vi "加标回收调试界面.vi"() -> ()   [LabVIEW 2016, in "质控单元V2.lvlib"]
uses:
  <vilib>/Utility/miscctls.llb/LVPointTypeDef.ctl
  <vilib>/Utility/miscctls.llb/LVPositionTypeDef.ctl
panel:
  in  "关闭":bool
  out "流程 2":T1 {"进样流程"."进样流程-进样"."步骤二："."功能" items=["加标", "进样", "排液", "搅拌", "定量", "延时"]; "进样流程"."进样流程-进样"."步骤一："."功能" items=["加标", "进样", "排液", "搅拌", "定量", "延时"]; "进样流程"."进样流程-进样"."步骤四："."功能" items=["加标", "进样", "排液", "搅拌", "定量", "延时"]; "进样流程"."进样流程-进样"."步骤三："."功能" items=["加标", "进样", "排液", "搅拌", "定量", "延时"]; "进样流程"."进样流程-进样"."步骤六："."功能" items=["加标", "进样", "排液", "搅拌", "定量", "延时"]; "进样流程"."进样流程-进样"."步骤五："."功能" items=["加标", "进样", "排液", "搅拌", "定量", "延时"]; "进样流程"."进样流程-进样"."步骤八："."功能" items=["加标", "进样", "排液", "搅拌", "定量", "延时"]; "进样流程"."进样流程-进样"."步骤七："."功能" items=["加标", "进样", "排液", "搅拌", "定量", "延时"]; "进样流程"."进样流程-进样"."步骤十："."功能" items=["加标", "进样", "排液", "搅拌", "定量", "延时"]; "进样流程"."进样流程-进样"."步骤九："."功能" items=["加标", "进样", "排液", "搅拌", "定量", "延时"]; "进样流程"."进样流程-润洗"."步骤二："."功能" items=["加标", "进样", "排液", "搅拌", "定量", "延时"]; "进样流程"."进样流程-润洗"."步骤一："."功能" items=["加标", "进样", "排液", "搅拌", "定量", "延时"]; "进样流程"."进样流程-润洗"."步骤四："."功能" items=["加标", "进样", "排液", "搅拌", "定量", "延时"]; "进样流程"."进样流程-润洗"."步骤三："."功能" items=["加标", "进样", "排液", "搅拌", "定量", "延时"]; "进样流程"."进样流程-润洗"."步骤六："."功能" items=["加标", "进样", "排液", "搅拌", "定量", "延时"]; "进样流程"."进样流程-润洗"."步骤五："."功能" items=["加标", "进样", "排液", "搅拌", "定量", "延时"]; "进样流程"."进样流程-润洗"."步骤八："."功能" items=["加标", "进样", "排液", "搅拌", "定量", "延时"]; "进样流程"."进样流程-润洗"."步骤七："."功能" items=["加标", "进样", "排液", "搅拌", "定量", "延时"]; "进样流程"."进样流程-润洗"."步骤十："."功能" items=["加标", "进样", "排液", "搅拌", "定量", "延时"]; "进样流程"."进样流程-润洗"."步骤九："."功能" items=["加标", "进样", "排液", "搅拌", "定量", "延时"]; "排液流程"."步骤二："."功能" items=["加标", "进样", "排液", "搅拌", "定量", "延时"]; "排液流程"."步骤一："."功能" items=["加标", "进样", "排液", "搅拌", "定量", "延时"]; "排液流程"."步骤四："."功能" items=["加标", "进样", "排液", "搅拌", "定量", "延时"]; "排液流程"."步骤三："."功能" items=["加标", "进样", "排液", "搅拌", "定量", "延时"]; "排液流程"."步骤六："."功能" items=["加标", "进样", "排液", "搅拌", "定量", "延时"]; "排液流程"."步骤五："."功能" items=["加标", "进样", "排液", "搅拌", "定量", "延时"]; "排液流程"."步骤八："."功能" items=["加标", "进样", "排液", "搅拌", "定量", "延时"]; "排液流程"."步骤七："."功能" items=["加标", "进样", "排液", "搅拌", "定量", "延时"]; "排液流程"."步骤十："."功能" items=["加标", "进样", "排液", "搅拌", "定量", "延时"]; "排液流程"."步骤九："."功能" items=["加标", "进样", "排液", "搅拌", "定量", "延时"]; "加标流程"."加标流程-加标"."步骤二："."功能" items=["加标", "进样", "排液", "搅拌", "定量", "延时"]; "加标流程"."加标流程-加标"."步骤一："."功能" items=["加标", "进样", "排液", "搅拌", "定量", "延时"]; "加标流程"."加标流程-加标"."步骤四："."功能" items=["加标", "进样", "排液", "搅拌", "定量", "延时"]; "加标流程"."加标流程-加标"."步骤三："."功能" items=["加标", "进样", "排液", "搅拌", "定量", "延时"]; "加标流程"."加标流程-加标"."步骤六："."功能" items=["加标", "进样", "排液", "搅拌", "定量", "延时"]; "加标流程"."加标流程-加标"."步骤五："."功能" items=["加标", "进样", "排液", "搅拌", "定量", "延时"]; "加标流程"."加标流程-加标"."步骤八："."功能" items=["加标", "进样", "排液", "搅拌", "定量", "延时"]; "加标流程"."加标流程-加标"."步骤七："."功能" items=["加标", "进样", "排液", "搅拌", "定量", "延时"]; "加标流程"."加标流程-加标"."步骤十："."功能" items=["加标", "进样", "排液", "搅拌", "定量", "延时"]; "加标流程"."加标流程-加标"."步骤九："."功能" items=["加标", "进样", "排液", "搅拌", "定量", "延时"]; "加标流程"."加标流程-定量"."步骤二："."功能" items=["加标", "进样", "排液", "搅拌", "定量", "延时"]; "加标流程"."加标流程-定量"."步骤一："."功能" items=["加标", "进样", "排液", "搅拌", "定量", "延时"]; "加标流程"."加标流程-定量"."步骤四："."功能" items=["加标", "进样", "排液", "搅拌", "定量", "延时"]; "加标流程"."加标流程-定量"."步骤三："."功能" items=["加标", "进样", "排液", "搅拌", "定量", "延时"]; "加标流程"."加标流程-定量"."步骤六："."功能" items=["加标", "进样", "排液", "搅拌", "定量", "延时"]; "加标流程"."加标流程-定量"."步骤五："."功能" items=["加标", "进样", "排液", "搅拌", "定量", "延时"]; "加标流程"."加标流程-定量"."步骤八："."功能" items=["加标", "进样", "排液", "搅拌", "定量", "延时"]; "加标流程"."加标流程-定量"."步骤七："."功能" items=["加标", "进样", "排液", "搅拌", "定量", "延时"]; "加标流程"."加标流程-定量"."步骤十："."功能" items=["加标", "进样", "排液", "搅拌", "定量", "延时"]; "加标流程"."加标流程-定量"."步骤九："."功能" items=["加标", "进样", "排液", "搅拌", "定量", "延时"]; "加标流程"."加标流程-进样"."步骤二："."功能" items=["加标", "进样", "排液", "搅拌", "定量", "延时"]; "加标流程"."加标流程-进样"."步骤一："."功能" items=["加标", "进样", "排液", "搅拌", "定量", "延时"]; "加标流程"."加标流程-进样"."步骤四："."功能" items=["加标", "进样", "排液", "搅拌", "定量", "延时"]; "加标流程"."加标流程-进样"."步骤三："."功能" items=["加标", "进样", "排液", "搅拌", "定量", "延时"]; "加标流程"."加标流程-进样"."步骤六："."功能" items=["加标", "进样", "排液", "搅拌", "定量", "延时"]; "加标流程"."加标流程-进样"."步骤五："."功能" items=["加标", "进样", "排液", "搅拌", "定量", "延时"]; "加标流程"."加标流程-进样"."步骤八："."功能" items=["加标", "进样", "排液", "搅拌", "定量", "延时"]; "加标流程"."加标流程-进样"."步骤七："."功能" items=["加标", "进样", "排液", "搅拌", "定量", "延时"]; "加标流程"."加标流程-进样"."步骤十："."功能" items=["加标", "进样", "排液", "搅拌", "定量", "延时"]; "加标流程"."加标流程-进样"."步骤九："."功能" items=["加标", "进样", "排液", "搅拌", "定量", "延时"]; "加标流程"."加标流程-润洗"."步骤二："."功能" items=["加标", "进样", "排液", "搅拌", "定量", "延时"]; "加标流程"."加标流程-润洗"."步骤一："."功能" items=["加标", "进样", "排液", "搅拌", "定量", "延时"]; "加标流程"."加标流程-润洗"."步骤四："."功能" items=["加标", "进样", "排液", "搅拌", "定量", "延时"]; "加标流程"."加标流程-润洗"."步骤三："."功能" items=["加标", "进样", "排液", "搅拌", "定量", "延时"]; "加标流程"."加标流程-润洗"."步骤六："."功能" items=["加标", "进样", "排液", "搅拌", "定量", "延时"]; "加标流程"."加标流程-润洗"."步骤五："."功能" items=["加标", "进样", "排液", "搅拌", "定量", "延时"]; "加标流程"."加标流程-润洗"."步骤八："."功能" items=["加标", "进样", "排液", "搅拌", "定量", "延时"]; "加标流程"."加标流程-润洗"."步骤七："."功能" items=["加标", "进样", "排液", "搅拌", "定量", "延时"]; "加标流程"."加标流程-润洗"."步骤十："."功能" items=["加标", "进样", "排液", "搅拌", "定量", "延时"]; "加标流程"."加标流程-润洗"."步骤九："."功能" items=["加标", "进样", "排液", "搅拌", "定量", "延时"]}
  in  "请选择模块":T2(radio)=enum."氨氮"
  in  "关于":bool
  in  "Tab Control 4":enum32{"参数"}(tab)
  out "剩余时间":string
  out "当前步骤":string
  out "当前流程":string
  out "告警状态":string
  out "液位状态":string
  out "运行状态":string
  out "通讯状态":bool caption="状态"
  in  "Tab Control 3":enum32{"参数设置", "单步调试", "流程写入"}(tab)
  in  "加标体积读取":bool
  in  "加标体积写入":bool
  in  "蠕动泵参数读取":bool
  in  "蠕动泵参数写入":bool
  in  "B":sgl
  in  "K":sgl
  in  "蠕动泵最小频率(Hz)":sgl
  in  "蠕动泵最大频率(Hz)":sgl
  in  "加标体积(mL)":sgl
  in  "注射泵系数读取":bool
  in  "注射泵系数写入":bool
  in  "蠕动泵2停止":bool
  in  "蠕动泵2正转":bool
  in  "蠕动泵2反转":bool
  in  "蠕动泵1停止":bool
  in  "蠕动泵1正转":bool
  in  "蠕动泵1反转":bool
  in  "三通阀2打开":bool
  in  "三通阀2关闭":bool
  in  "三通阀1打开":bool
  in  "三通阀1关闭":bool
  in  "注射泵复位":bool
  in  "注射泵暂停":bool
  in  "注射泵注入量":sgl=1000.0 min=0 max=1000 format="%u μL"
  in  "注射泵注出量":sgl=1000.0 min=0 max=1000 format="%u μL"
  in  "注射泵注出":bool
  in  "注射泵注入":bool
  in  "三通阀打开":bool
  in  "三通阀关闭":bool
  in  "流程保存":bool
  in  "流程加载":bool
  in  "流程写入":bool
  in  "流程读取":bool
  in  "子流程":u16(ring) items=["润洗"]
  in  "主流程":enum16{"进样流程", "加标流程", "排液流程"}(ring)
  in  "流程":T3 {"步骤二："."功能" items=["加标", "进样", "排液", "搅拌", "定量", "延时"]; "步骤四："."功能" items=["加标", "进样", "排液", "搅拌", "定量", "延时"]; "步骤六："."功能" items=["加标", "进样", "排液", "搅拌", "定量", "延时"]; "步骤八："."功能" items=["加标", "进样", "排液", "搅拌", "定量", "延时"]; "步骤十："."功能" items=["加标", "进样", "排液", "搅拌", "定量", "延时"]; "步骤一："."功能" items=["加标", "进样", "排液", "搅拌", "定量", "延时"]; "步骤三："."功能" items=["加标", "进样", "排液", "搅拌", "定量", "延时"]; "步骤五："."功能" items=["加标", "进样", "排液", "搅拌", "定量", "延时"]; "步骤七："."功能" items=["加标", "进样", "排液", "搅拌", "定量", "延时"]; "步骤九："."功能" items=["加标", "进样", "排液", "搅拌", "定量", "延时"]}
  in  "Tab Control 2":enum32{"参数"}(tab)
  in  "组合操作加标":bool
  in  "启动进样流程":bool
  in  "启动加标流程":bool
  in  "启动排液流程":bool
  in  "停止所有流程":bool
  in  "组合操作停止":bool
  in  "组合操作定量":bool
  in  "组合操作进空气":bool
  in  "组合操作排废液":bool
  in  "组合操作进水样":bool
  in  "清除告警":bool
  in  "加标体积输入":sgl=0.1 min=0 max=1000 format="%#.4f mL"
  # "仪器状态"
  # "柱塞泵泵系数"
  # "柱塞泵"
  # "三通阀"
  # "泵阀"
  # "三通阀1"
  # "三通阀2"
  # "蠕动泵1"
  # "蠕动泵2"
  # "仪器端："
  # "PC端："
  # "组合步骤"
  # "测试流程"
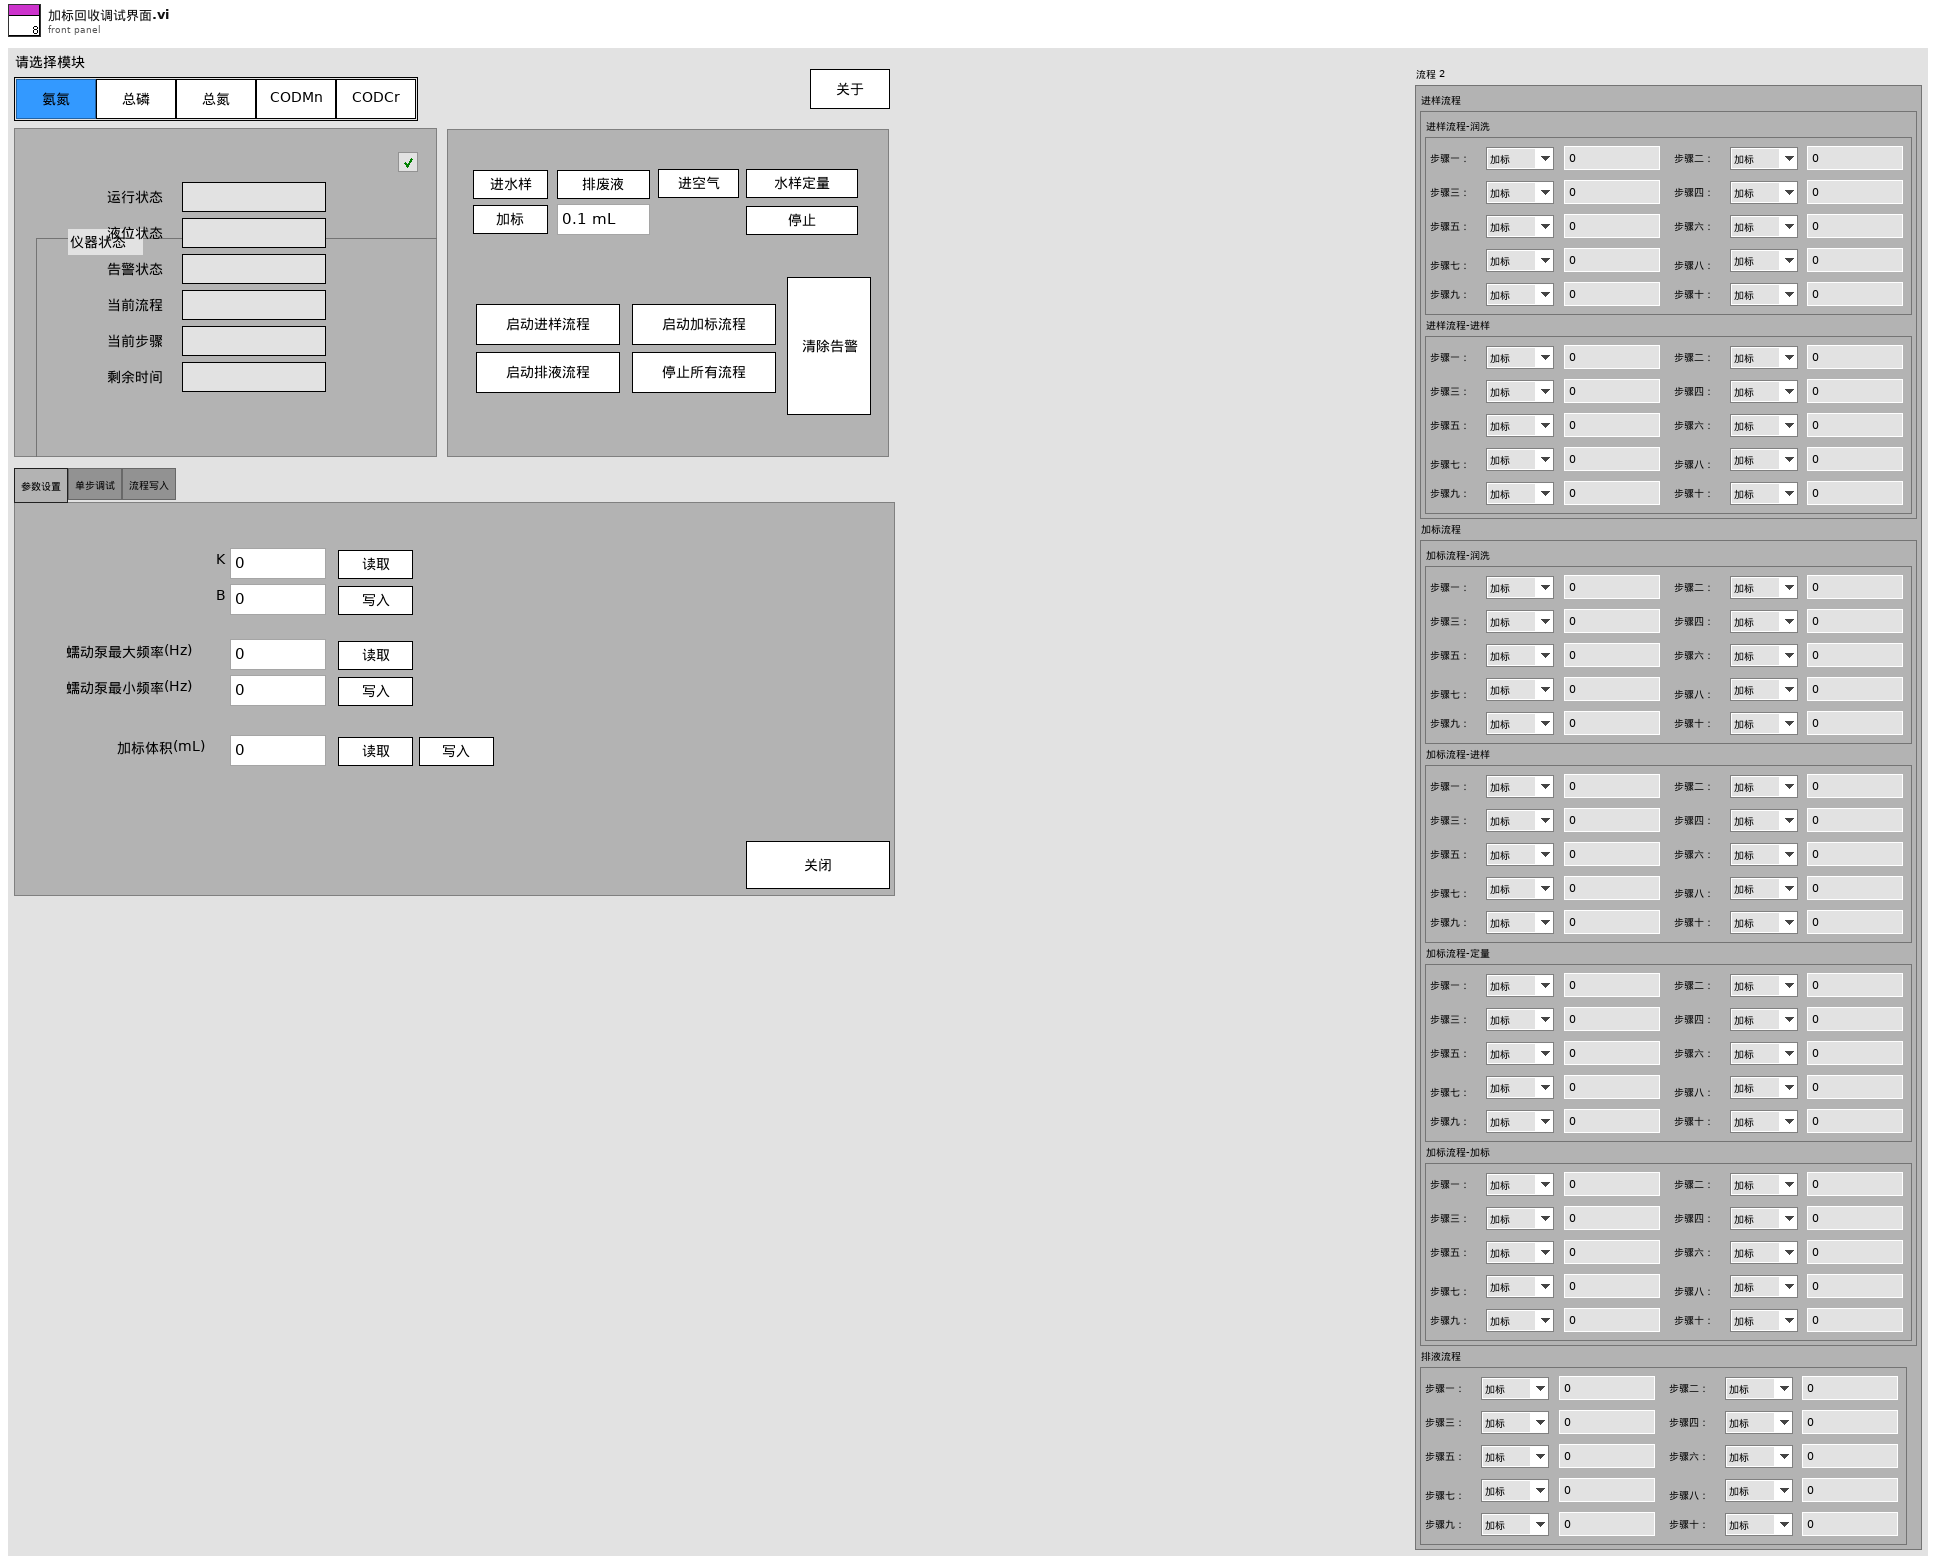
[diagram p1: front panel]
types:
  T1 = cluster{"进样流程":cluster{"进样流程-润洗":cluster{"步骤一：":cluster{"功能":u16, "值":sgl}, "步骤二：":cluster{"功能":u16, "值":sgl}, "步骤三：":cluster{"功能":u16, "值":sgl}, "步骤四：":cluster{"功能":u16, "值":sgl}, "步骤五：":cluster{"功能":u16, "值":sgl}, "步骤六：":cluster{"功能":u16, "值":sgl}, "步骤七：":cluster{"功能":u16, "值":sgl}, "步骤八：":cluster{"功能":u16, "值":sgl}, "步骤九：":cluster{"功能":u16, "值":sgl}, "步骤十：":cluster{"功能":u16, "值":sgl}}, "进样流程-进样":cluster{"步骤一：":cluster{"功能":u16, "值":sgl}, "步骤二：":cluster{"功能":u16, "值":sgl}, "步骤三：":cluster{"功能":u16, "值":sgl}, "步骤四：":cluster{"功能":u16, "值":sgl}, "步骤五：":cluster{"功能":u16, "值":sgl}, "步骤六：":cluster{"功能":u16, "值":sgl}, "步骤七：":cluster{"功能":u16, "值":sgl}, "步骤八：":cluster{"功能":u16, "值":sgl}, "步骤九：":cluster{"功能":u16, "值":sgl}, "步骤十：":cluster{"功能":u16, "值":sgl}}}, "加标流程":cluster{"加标流程-润洗":cluster{"步骤一：":cluster{"功能":u16, "值":sgl}, "步骤二：":cluster{"功能":u16, "值":sgl}, "步骤三：":cluster{"功能":u16, "值":sgl}, "步骤四：":cluster{"功能":u16, "值":sgl}, "步骤五：":cluster{"功能":u16, "值":sgl}, "步骤六：":cluster{"功能":u16, "值":sgl}, "步骤七：":cluster{"功能":u16, "值":sgl}, "步骤八：":cluster{"功能":u16, "值":sgl}, "步骤九：":cluster{"功能":u16, "值":sgl}, "步骤十：":cluster{"功能":u16, "值":sgl}}, "加标流程-进样":cluster{"步骤一：":cluster{"功能":u16, "值":sgl}, "步骤二：":cluster{"功能":u16, "值":sgl}, "步骤三：":cluster{"功能":u16, "值":sgl}, "步骤四：":cluster{"功能":u16, "值":sgl}, "步骤五：":cluster{"功能":u16, "值":sgl}, "步骤六：":cluster{"功能":u16, "值":sgl}, "步骤七：":cluster{"功能":u16, "值":sgl}, "步骤八：":cluster{"功能":u16, "值":sgl}, "步骤九：":cluster{"功能":u16, "值":sgl}, "步骤十：":cluster{"功能":u16, "值":sgl}}, "加标流程-定量":cluster{"步骤一：":cluster{"功能":u16, "值":sgl}, "步骤二：":cluster{"功能":u16, "值":sgl}, "步骤三：":cluster{"功能":u16, "值":sgl}, "步骤四：":cluster{"功能":u16, "值":sgl}, "步骤五：":cluster{"功能":u16, "值":sgl}, "步骤六：":cluster{"功能":u16, "值":sgl}, "步骤七：":cluster{"功能":u16, "值":sgl}, "步骤八：":cluster{"功能":u16, "值":sgl}, "步骤九：":cluster{"功能":u16, "值":sgl}, "步骤十：":cluster{"功能":u16, "值":sgl}}, "加标流程-加标":cluster{"步骤一：":cluster{"功能":u16, "值":sgl}, "步骤二：":cluster{"功能":u16, "值":sgl}, "步骤三：":cluster{"功能":u16, "值":sgl}, "步骤四：":cluster{"功能":u16, "值":sgl}, "步骤五：":cluster{"功能":u16, "值":sgl}, "步骤六：":cluster{"功能":u16, "值":sgl}, "步骤七：":cluster{"功能":u16, "值":sgl}, "步骤八：":cluster{"功能":u16, "值":sgl}, "步骤九：":cluster{"功能":u16, "值":sgl}, "步骤十：":cluster{"功能":u16, "值":sgl}}}, "排液流程":cluster{"步骤一：":cluster{"功能":u16, "值":sgl}, "步骤二：":cluster{"功能":u16, "值":sgl}, "步骤三：":cluster{"功能":u16, "值":sgl}, "步骤四：":cluster{"功能":u16, "值":sgl}, "步骤五：":cluster{"功能":u16, "值":sgl}, "步骤六：":cluster{"功能":u16, "值":sgl}, "步骤七：":cluster{"功能":u16, "值":sgl}, "步骤八：":cluster{"功能":u16, "值":sgl}, "步骤九：":cluster{"功能":u16, "值":sgl}, "步骤十：":cluster{"功能":u16, "值":sgl}}}
  T2 = enum32{"未选择", "氨氮", "总磷", "总氮", "CODMn", "CODCr", "氨氮总磷", "总磷总氮"}
  T3 = cluster{"步骤一：":cluster{"功能":u16, "值":sgl}, "步骤二：":cluster{"功能":u16, "值":sgl}, "步骤三：":cluster{"功能":u16, "值":sgl}, "步骤四：":cluster{"功能":u16, "值":sgl}, "步骤五：":cluster{"功能":u16, "值":sgl}, "步骤六：":cluster{"功能":u16, "值":sgl}, "步骤七：":cluster{"功能":u16, "值":sgl}, "步骤八：":cluster{"功能":u16, "值":sgl}, "步骤九：":cluster{"功能":u16, "值":sgl}, "步骤十：":cluster{"功能":u16, "值":sgl}}
  T4 = typedef "LVPositionTypeDef.ctl" = cluster{"Left":i32, "Top":i32}
  T5 = typedef "LVPointTypeDef.ctl" = cluster{"Horizontal":i16, "Vertical":i16}
  T6 = typedef "质控单元V2.lvlib/质控slave id.ctl" = enum16{"null", "氨氮", "总磷", "总氮", "CODMn", "CODCr"}
  T7 = typedef "质控单元V2.lvlib/质控注射泵操作.ctl" = enum16{"打开三通阀", "关闭三通阀", "注射泵吸入", "注射泵排出", "注射泵暂停", "注射泵复位"}
  T8 = typedef "质控单元V2.lvlib/质控组合命令区.ctl" = enum16{"停止", "进水样", "排废液", "进空气（搅拌）", "定量（反转定量）", "加标"}
  T9 = typedef "质控单元V2.lvlib/质控流程控制.ctl" = enum16{"待机", "启动进样流程", "启动加标流程", "启动排液流程", "停止流程", "加标（单独一步骤）"}
  T10 = typedef "质控单元V2.lvlib/质控仪器状态显示.ctl" = cluster{"运行模式":string, "运行状态":string, "液位状态":string, "告警状态":string, "当前流程":string, "当前步骤":string, "剩余时间":string}
  T11 = typedef "质控单元V2.lvlib/质控蠕动泵操作.ctl" = u16
  T12 = typedef "LVRectTypeDef.ctl" = cluster{"Left":i16, "Top":i16, "Right":i16, "Bottom":i16}
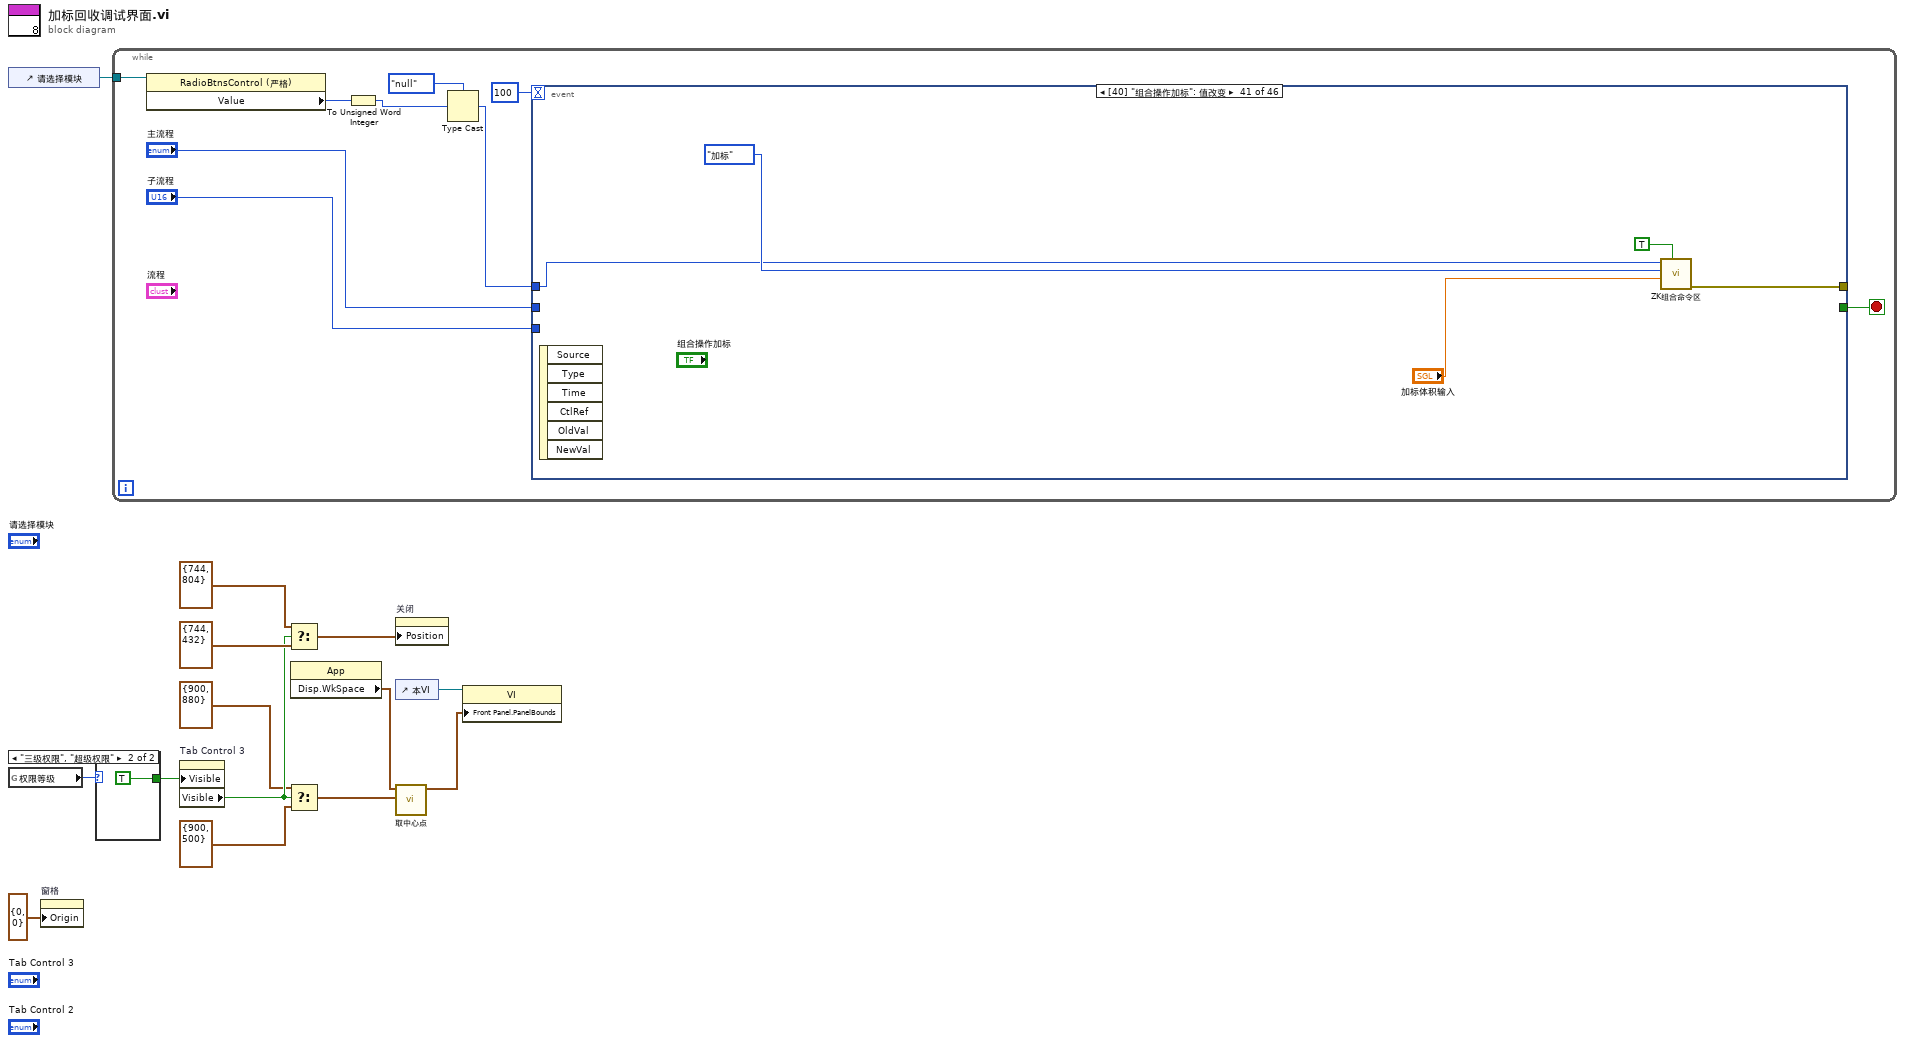
[diagram p0: block diagram]
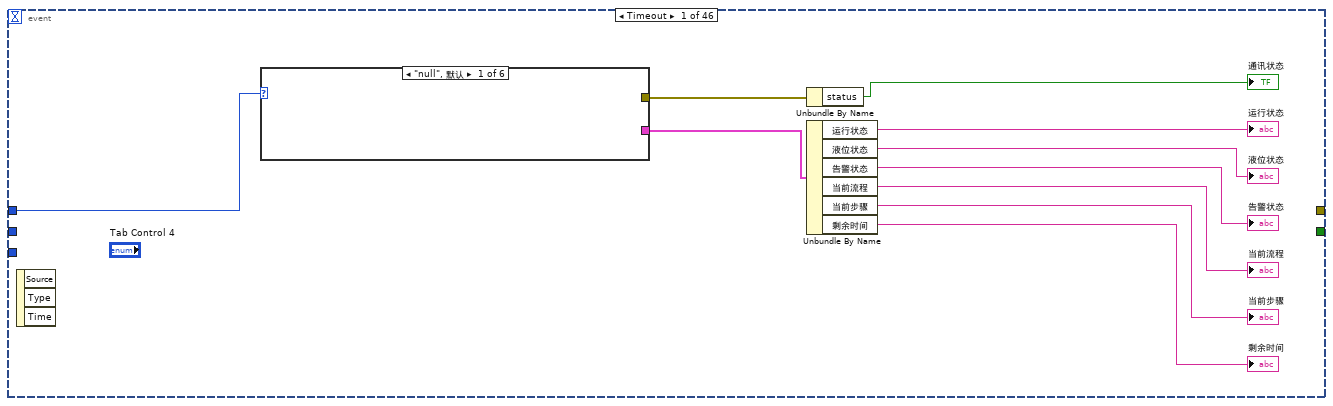
[diagram p3: hidden frame]
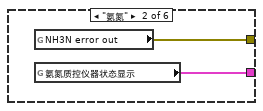
[diagram p4: hidden frame]
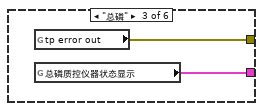
[diagram p5: hidden frame]
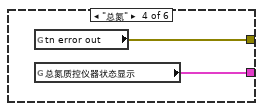
[diagram p6: hidden frame]
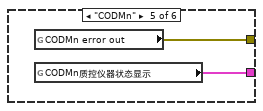
[diagram p7: hidden frame]
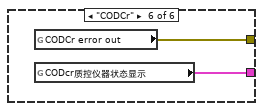
[diagram p8: hidden frame]
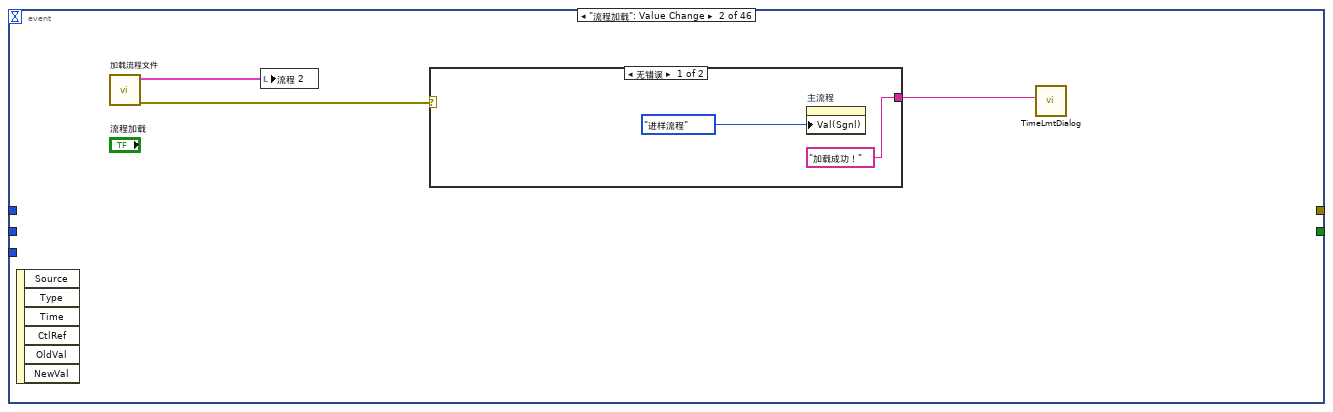
[diagram p9: hidden frame]
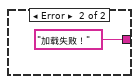
[diagram p10: hidden frame]
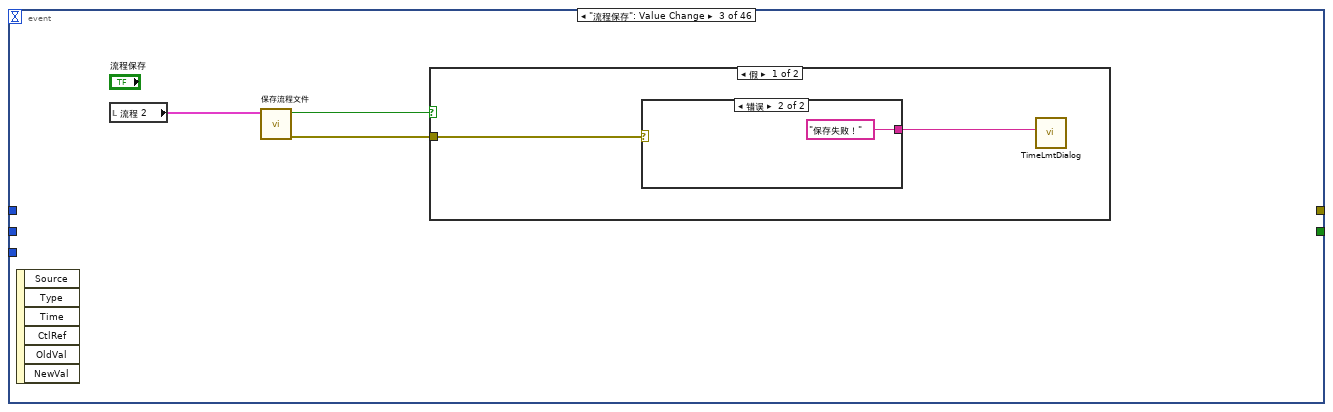
[diagram p11: hidden frame]
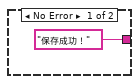
[diagram p12: hidden frame]
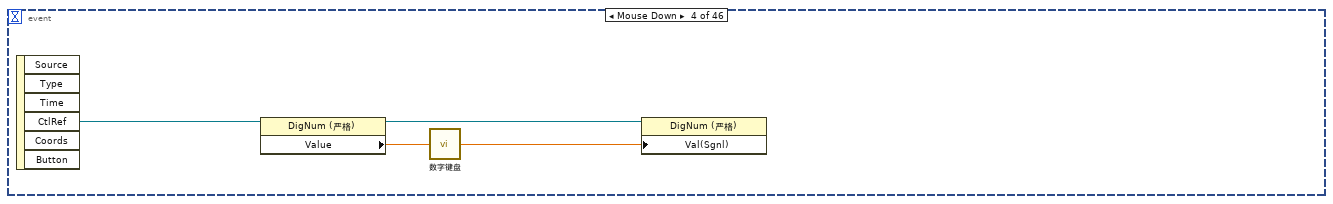
[diagram p14: hidden frame]
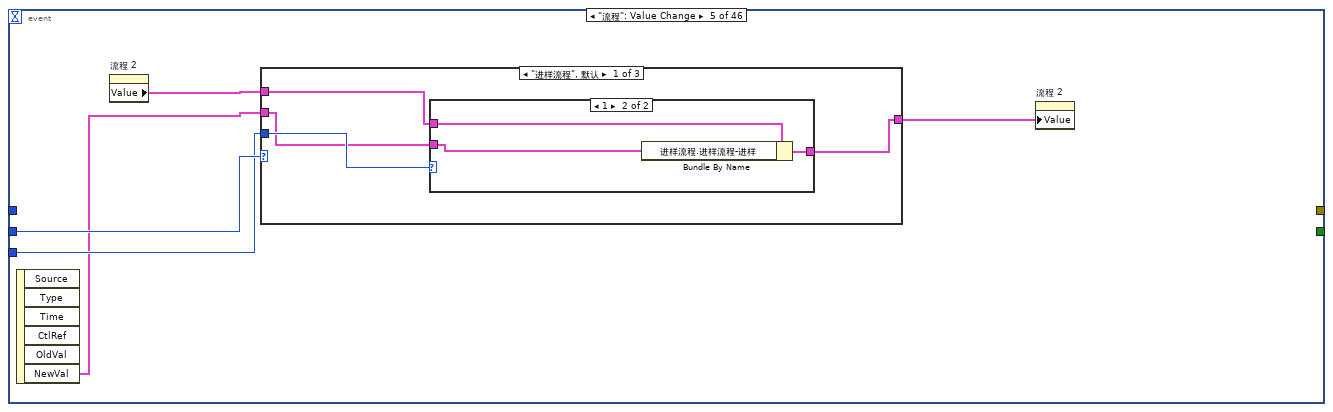
[diagram p15: hidden frame]
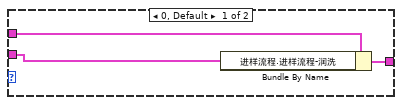
[diagram p16: hidden frame]
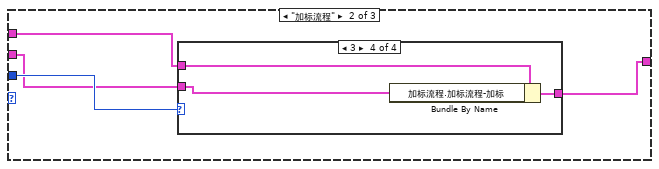
[diagram p17: hidden frame]
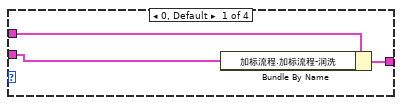
[diagram p18: hidden frame]
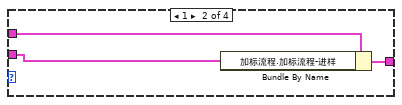
[diagram p19: hidden frame]
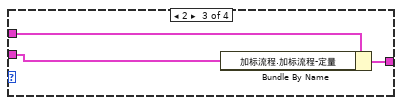
[diagram p20: hidden frame]
diagram:
  n1 = control-ref of="请选择模块"() -> (w13:refnum<vi>)
  n2 = global read "ZK非断电保存全局变量.vi" "权限等级"() -> (w2:enum16{"一级权限", "二级权限", "三级权限", "超级权限"})
  n3 = property on="窗格" class="Pane"("Origin"=T5 {"Horizontal"=0, "Vertical"=0} ("原点")) -> ()  [unwired: 2 in, 2 out]
  n4 = case shown="\"三级权限\", \"超级权限\"" w2 {
    tunnel: [_ TRUE] -> w1
    frame "一级权限", Default {
    }
    frame "三级权限", "超级权限" {
    }
  }
  n5 = while {
    tunnel: w13 -> [w22]
    stop <- w24 stop-if-true
    n6 = property class="RadioBtnsControl (严格)"(reference=w22) -> ("Value"=w19:T2)  [unwired: 1 in, 2 out]
    n7 = To Unsigned Word Integer(number=w19) -> (unsigned 16bit integer=w18:u16)
    n8 = Type Cast(type=质控slave_id."null" ("请选择模块"), x=w18) -> (*(type *) &x=w20:T6)
    n9 = event shown="[40] \"组合操作加标\": 值改变" {
      selector: _ -> [_ _ _ _ _ _ _ _ _ _ _ _ _ _ _ _ _ _ _ _ _ _ _ _ _ _ _ _ _ _ _ _ _ _ _ _ _ _ _ _ _ _ _ _ _ _]
      dyn-events: _ -> [_ _ _ _ _ _ _ _ _ _ _ _ _ _ _ _ _ _ _ _ _ _ _ _ _ _ _ _ _ _ _ _ _ _ _ _ _ _ _ _ _ _ _ _ _ _]
      timeout: 100 -> [_ _ _ _ _ _ _ _ _ _ _ _ _ _ _ _ _ _ _ _ _ _ _ _ _ _ _ _ _ _ _ _ _ _ _ _ _ _ _ _ _ _ _ _ _ _]
      tunnel: [_ _ _ _ _ _ _ _ _ _ _ TRUE _ _ _ _ _ _ _ _ _ _ _ _ _ _ _ _ _ _ _ _ _ _ _ _ _ _ _ _ _ _ _ _ _ _] -> w24
      tunnel: [_ _ _ _ _ _ _ _ _ _ w160 _ _ _ w174 w179 w186 w189 w195 w199 w202 w207 w217 w227 w231 w235 w238 w242 w246 w250 w255 w259 w263 w267 w271 w275 w279 w283 w287 w291 w296 w300 w304 w308 w312 w316] -> _
      tunnel: w20 -> [w27 _ _ _ _ w99 w102 _ _ w157 w158 _ _ _ w172 w177 w182 w187 w192 w196 w200 w204 w210 w221 w228 w232 w236 w240 w244 w248 w252 w256 w260 w264 w268 w272 w276 w280 w284 w288 w293 w297 w301 w305 w309 w313]
      tunnel: "子流程" -> [_ _ _ _ w64 _ _ w108 _ _ _ _ _ _ _ _ _ _ _ _ _ _ _ _ _ _ _ _ _ _ _ _ _ _ _ _ _ _ _ _ _ _ _ _ _ _]
      tunnel: "主流程" -> [_ _ _ _ w65 _ _ _ w134 _ _ _ _ _ _ _ _ _ _ _ _ _ _ _ _ _ _ _ _ _ _ _ _ _ _ _ _ _ _ _ _ _ _ _ _ _]
      event Timeout {
        n10 = event-data() -> ()  [unwired: 1 in, 3 out]
        n11 = case shown="\"null\", 默认" w27 {
          tunnel: [_ w36 w38 w40 w42 w44] -> w34
          tunnel: [_ w35 w37 w39 w41 w43] -> w26
          frame "null", Default {
          }
          frame "氨氮" {
            n12 = global read "ZK非断电保存全局变量.vi" "NH3N error out"() -> (w35:errorcluster)
            n13 = global read "ZK非断电保存全局变量.vi" "氨氮质控仪器状态显示"() -> (w36:T10)
          }
          frame "总磷" {
            n14 = global read "ZK非断电保存全局变量.vi" "tp error out"() -> (w37:errorcluster)
            n15 = global read "ZK非断电保存全局变量.vi" "总磷质控仪器状态显示"() -> (w38:T10)
          }
          frame "总氮" {
            n16 = global read "ZK非断电保存全局变量.vi" "tn error out"() -> (w39:errorcluster)
            n17 = global read "ZK非断电保存全局变量.vi" "总氮质控仪器状态显示"() -> (w40:T10)
          }
          frame "CODMn" {
            n18 = global read "ZK非断电保存全局变量.vi" "CODMn error out"() -> (w41:errorcluster)
            n19 = global read "ZK非断电保存全局变量.vi" "CODMn质控仪器状态显示"() -> (w42:T10)
          }
          frame "CODCr" {
            n20 = global read "ZK非断电保存全局变量.vi" "CODCr error out"() -> (w43:errorcluster)
            n21 = global read "ZK非断电保存全局变量.vi" "CODcr质控仪器状态显示"() -> (w44:T10)
          }
        }
        n22 = Unbundle By Name(w26) -> ("status"=→"通讯状态":bool)
        n23 = Unbundle By Name(w34) -> ("运行状态"=→"运行状态":string, "液位状态"=→"液位状态":string, "告警状态"=→"告警状态":string, "当前流程"=→"当前流程":string, "当前步骤"=→"当前步骤":string, "剩余时间"=→"剩余时间":string)
      }
      event "流程加载": Value Change {
        n24 = event-data() -> ()  [unwired: 1 in, 6 out]
        n25 = call "加载流程文件.vi"() -> ("错误输出"=w46:errorcluster, "流程"=w47:T1)  [unwired: 10 in]
        n26 = local write "流程 2"(w47) -> ()
        n27 = case shown="无错误" w46 {
          tunnel: ["加载成功！" "加载失败！"] -> w45
          frame No Error {
            n28 = property on="主流程" class="Enum (严格)"("Val(Sgnl)"=enum16{"进样流程", "加标流程", "排液流程"}."进样流程" ("值(信号)")) -> ()  [unwired: 2 in, 2 out]
          }
          frame Error {
          }
        }
        n29 = call "TimeLmtDialog.vi"("Infoin"=w45) -> ()  [unwired: 11 in]
      }
      event "流程保存": Value Change {
        n30 = event-data() -> ()  [unwired: 1 in, 6 out]
        n31 = local read "流程 2"() -> (w53:T1)
        n32 = call "保存流程文件.vi"("流程"=w53) -> ("错误输出"=w52:errorcluster, "cancelled"=w51:bool)  [unwired: 9 in]
        n33 = case shown="假" w51 {
          tunnel: w52 -> [w54 _]
          frame False {
            n34 = case shown="错误" w54 {
              tunnel: ["保存成功！" "保存失败！"] -> w55
              frame No Error {
              }
              frame Error {
              }
            }
            n35 = call "TimeLmtDialog.vi"("Infoin"=w55) -> ()  [unwired: 11 in]
          }
          frame True {
          }
        }
      }
      event "流程.步骤一：.值", "流程.步骤二：.值", "流程.步骤三：.值", "流程.步骤四：.值", "流程.步骤五：.值", "流程.步骤六：.值", "流程.步骤七：.值", "流程.步骤八：.值", "流程.步骤九：.值", "流程.步骤十：.值": Mouse Down {
        n36 = event-data() -> ("CtlRef"=w58:refnum<vi>)  [unwired: 1 in, 5 out]
        n37 = property class="DigNum (严格)"(reference=w58) -> (reference out=w61:refnum<vi>, "Value"=w59:sgl)  [unwired: 1 in, 1 out]
        n38 = call "数字键盘.vi"("OldNumber"=w59) -> ("NewNumber"=w60:sgl)
        n39 = property class="DigNum (严格)"(reference=w61, "Val(Sgnl)"=w60) -> ()  [unwired: 1 in, 2 out]
      }
      event "流程": Value Change {
        n40 = event-data() -> ("NewVal"=w63:T3)  [unwired: 1 in, 5 out]
        n41 = property on="流程 2" class="Clust (严格)"() -> ("Value"=w66:T1)  [unwired: 2 in, 2 out]
        n42 = case shown="\"进样流程\", 默认" w65 {
          tunnel: w66 -> [w69 w79 w95]
          tunnel: w64 -> [w70 w80 _]
          tunnel: w63 -> [w68 w77 w94]
          tunnel: [w67 w78 w93] -> w62
          frame "进样流程", Default {
            n43 = case shown="1" w70 {
              tunnel: w69 -> [w73 w76]
              tunnel: w68 -> [w72 w75]
              tunnel: [w71 w74] -> w67
              frame 0, Default {
                n44 = Bundle By Name(cluster=w73, "进样流程.进样流程-润洗"=w72) -> (w71:T1)
              }
              frame 1 {
                n45 = Bundle By Name(cluster=w76, "进样流程.进样流程-进样"=w75) -> (w74:T1)
              }
            }
          }
          frame "加标流程" {
            n46 = case shown="3" w80 {
              tunnel: w79 -> [w83 w86 w88 w92]
              tunnel: [w82 w84 w87 w90] -> w78
              tunnel: w77 -> [w81 w85 w89 w91]
              frame 0, Default {
                n47 = Bundle By Name(cluster=w83, "加标流程.加标流程-润洗"=w81) -> (w82:T1)
              }
              frame 1 {
                n48 = Bundle By Name(cluster=w86, "加标流程.加标流程-进样"=w85) -> (w84:T1)
              }
              frame 2 {
                n49 = Bundle By Name(cluster=w88, "加标流程.加标流程-定量"=w89) -> (w87:T1)
              }
              frame 3 {
                n50 = Bundle By Name(cluster=w92, "加标流程.加标流程-加标"=w91) -> (w90:T1)
              }
            }
          }
          frame "排液流程" {
            n51 = Bundle By Name(cluster=w95, "排液流程"=w94) -> (w93:T1)
          }
        }
        n52 = property on="流程 2" class="Clust (严格)"("Value"=w62) -> ()  [unwired: 2 in, 2 out]
      }
      event "流程读取": Value Change {
        n53 = event-data() -> ()  [unwired: 1 in, 6 out]
        n54 = call "ZK流程读取.vi"("是否启用通讯通知"=TRUE, "Slave ID"=w99) -> ("error out"=w96:errorcluster, "流程"=→"流程 2":T1)  [unwired: 8 in]
        n55 = case shown="无错误" w96 {
          frame No Error {
            n56 = property on="主流程" class="Enum (严格)"("Val(Sgnl)"=enum16{"进样流程", "加标流程", "排液流程"}."进样流程" ("值(信号)")) -> ()  [unwired: 2 in, 2 out]
          }
          frame Error {
          }
        }
      }
      event "流程写入": Value Change {
        n57 = event-data() -> ()  [unwired: 1 in, 6 out]
        n58 = property on="流程 2" class="Clust (严格)"() -> ("Value"=w103:T1)  [unwired: 2 in, 2 out]
        n59 = call "ZK流程写入.vi"("是否启用通讯通知"=TRUE, "流程"=w103, "Slave ID"=w102) -> ()  [unwired: 8 in, 1 out]
      }
      event "主流程": Value Change {
        n60 = event-data() -> ("NewVal"=w104:enum16{"进样流程", "加标流程", "排液流程"})  [unwired: 1 in, 5 out]
        n61 = local read "流程 2"() -> (w109:T1)
        n62 = case shown="\"进样流程\", 默认" w104 {
          tunnel: w109 -> [w112 w120 w132]
          tunnel: w108 -> [w113 w121 _]
          tunnel: [w111 w119 w131] -> w107
          tunnel: [string[] ["润洗", "进样"] ("字符串[]") string[] ["润洗", "进样", "定量", "加标"] ("字符串[]") string[] ["排液"] ("字符串[]")] -> w106
          frame "进样流程", Default {
            n63 = case shown="0, 默认" w113 {
              tunnel: w112 -> [w115 w117]
              tunnel: [w114 w116] -> w111
              frame 0, Default {
                n64 = Unbundle By Name(w115) -> ("进样流程.进样流程-润洗"=w114:T3)
              }
              frame 1 {
                n65 = Unbundle By Name(w117) -> ("进样流程.进样流程-进样"=w116:T3)
              }
            }
          }
          frame "加标流程" {
            n66 = case shown="3" w121 {
              tunnel: w120 -> [w123 w125 w127 w129]
              tunnel: [w122 w124 w126 w128] -> w119
              frame 0, Default {
                n67 = Unbundle By Name(w123) -> ("加标流程.加标流程-润洗"=w122:T3)
              }
              frame 1 {
                n68 = Unbundle By Name(w125) -> ("加标流程.加标流程-进样"=w124:T3)
              }
              frame 2 {
                n69 = Unbundle By Name(w127) -> ("加标流程.加标流程-定量"=w126:T3)
              }
              frame 3 {
                n70 = Unbundle By Name(w129) -> ("加标流程.加标流程-加标"=w128:T3)
              }
            }
          }
          frame "排液流程" {
            n71 = Unbundle By Name(w132) -> ("排液流程"=w131:T3)
          }
        }
        n72 = local write "流程"(w107) -> ()
        n73 = property on="子流程" class="Ring (严格)"("Strings []"=w106, "Value"=0) -> ()  [unwired: 2 in, 2 out]
      }
      event "子流程": Value Change {
        n74 = event-data() -> ("NewVal"=w133:u16)  [unwired: 1 in, 5 out]
        n75 = local read "流程 2"() -> (w136:T1)
        n76 = case shown="\"进样流程\", 默认" w134 {
          tunnel: w136 -> [w138 w145 w156]
          tunnel: w133 -> [w139 w146 _]
          tunnel: [w137 w144 w155] -> w135
          frame "进样流程", Default {
            n77 = case shown="0, 默认" w139 {
              tunnel: w138 -> [w141 w143]
              tunnel: [w140 w142] -> w137
              frame 0, Default {
                n78 = Unbundle By Name(w141) -> ("进样流程.进样流程-润洗"=w140:T3)
              }
              frame 1 {
                n79 = Unbundle By Name(w143) -> ("进样流程.进样流程-进样"=w142:T3)
              }
            }
          }
          frame "加标流程" {
            n80 = case shown="3" w146 {
              tunnel: w145 -> [w148 w150 w152 w154]
              tunnel: [w147 w149 w151 w153] -> w144
              frame 0, Default {
                n81 = Unbundle By Name(w148) -> ("加标流程.加标流程-润洗"=w147:T3)
              }
              frame 1 {
                n82 = Unbundle By Name(w150) -> ("加标流程.加标流程-进样"=w149:T3)
              }
              frame 2 {
                n83 = Unbundle By Name(w152) -> ("加标流程.加标流程-定量"=w151:T3)
              }
              frame 3 {
                n84 = Unbundle By Name(w154) -> ("加标流程.加标流程-加标"=w153:T3)
              }
            }
          }
          frame "排液流程" {
            n85 = Unbundle By Name(w156) -> ("排液流程"=w155:T3)
          }
        }
        n86 = local write "流程"(w135) -> ()
      }
      event "关于": Value Change {
        n87 = event-data() -> ()  [unwired: 1 in, 6 out]
        n88 = call "质控关于.vi"("Slave ID"=w157) -> ()  [unwired: 11 in]
      }
      event "清除告警": Value Change {
        n89 = event-data() -> ()  [unwired: 1 in, 6 out]
        n90 = call "ZK报警清除.vi"("是否启用通讯通知"=TRUE, "Slave ID"=w158) -> ("error out"=w160:errorcluster)  [unwired: 9 in]
      }
      event Panel Close; "关闭": Value Change {
        n91 = event-data() -> ()  [unwired: 1 in, 3 out]
      }
      event "K", "B", "蠕动泵最小频率(Hz)", "蠕动泵最大频率(Hz)", "加标体积(mL)", "注射泵注出量", "注射泵注入量": Mouse Down {
        n92 = event-data() -> ("CtlRef"=w165:refnum<vi>)  [unwired: 1 in, 2 out]
        n93 = property class="DigNum (严格)"(reference=w165) -> (reference out=w164:refnum<vi>, "Value"=w162:sgl)  [unwired: 1 in, 1 out]
        n94 = call "数字键盘.vi"("OldNumber"=w162) -> ("NewNumber"=w163:sgl)
        n95 = property class="DigNum (严格)"(reference=w164, "Val(Sgnl)"=w163) -> ()  [unwired: 1 in, 2 out]
      }
      event "注射泵注出量", "注射泵注入量": Value Change {
        w167 = sgl 1000.0 ("y")
        n96 = event-data() -> ("CtlRef"=w168:refnum<vi>, "NewVal"=w169:sgl)  [unwired: 1 in, 4 out]
        n97 = Greater Or Equal?(x=w169, y=w167) -> (x >= y?=w166:bool)
        n98 = case shown="真" w166 {
          tunnel: w168 -> [_ w171]
          tunnel: w167 -> [_ w170]
          frame False {
          }
          frame True {
            n99 = property class="DigNum (严格)"(reference=w171, "Value"=w170) -> ()  [unwired: 1 in, 2 out]
          }
        }
      }
      event "注射泵系数读取": Value Change {
        n100 = event-data() -> ()  [unwired: 1 in, 4 out]
        n101 = call "ZK注射泵系数读取.vi"("是否启用通讯通知"=TRUE, "Slave ID"=w172) -> ("error out"=w174:errorcluster, "B"=w175:sgl, "K"=w176:sgl)  [unwired: 7 in]
        n102 = local write "K"(w176) -> ()
        n103 = local write "B"(w175) -> ()
      }
      event "注射泵系数写入": Value Change {
        n104 = event-data() -> ()  [unwired: 1 in, 4 out]
        n105 = call "ZK注射泵系数写入.vi"("是否启用通讯通知"=TRUE, "B"="B", "K"="K", "Slave ID"=w177) -> ("error out"=w179:errorcluster)  [unwired: 7 in]
      }
      event "蠕动泵参数写入": Value Change {
        n106 = event-data() -> ()  [unwired: 1 in, 5 out]
        n107 = call "ZK蠕动泵频率参数写入.vi"("是否启用通讯通知"=TRUE, "蠕动泵最小频率"="蠕动泵最小频率(Hz)", "蠕动泵最大频率"="蠕动泵最大频率(Hz)", "Slave ID"=w182) -> ("error out"=w186:errorcluster)  [unwired: 7 in]
      }
      event "蠕动泵参数读取": Value Change {
        n108 = event-data() -> ()  [unwired: 1 in, 5 out]
        n109 = call "ZK蠕动泵频率参数读取.vi"("是否启用通讯通知"=TRUE, "Slave ID"=w187) -> ("error out"=w189:errorcluster, "蠕动泵最小频率"=w190:i32, "蠕动泵最大频率"=w191:i32)  [unwired: 7 in]
        n110 = local write "蠕动泵最大频率(Hz)"(w191) -> ()
        n111 = local write "蠕动泵最小频率(Hz)"(w190) -> ()
      }
      event "加标体积写入": Value Change {
        n112 = event-data() -> ()  [unwired: 1 in, 6 out]
        n113 = call "ZK加标体积写入.vi"("是否启用通讯通知"=TRUE, "加标体积"="加标体积(mL)", "Slave ID"=w192) -> ("error out"=w195:errorcluster)  [unwired: 8 in]
      }
      event "加标体积读取": Value Change {
        n114 = event-data() -> ()  [unwired: 1 in, 6 out]
        n115 = call "ZK加标体积读取.vi"("是否启用通讯通知"=TRUE, "Slave ID"=w196) -> ("error out"=w199:errorcluster, "加标体积"=w198:sgl)  [unwired: 8 in]
        n116 = local write "加标体积(mL)"(w198) -> ()
      }
      event "三通阀打开": Value Change {
        n117 = event-data() -> ()  [unwired: 1 in, 6 out]
        n118 = call "ZK注射泵操作.vi"("是否启用通讯通知"=TRUE, "注射泵操作"=质控注射泵操作."打开三通阀", "Slave ID"=w200) -> ("error out"=w202:errorcluster)  [unwired: 8 in]
      }
      event "三通阀关闭": Value Change {
        n119 = event-data() -> ()  [unwired: 1 in, 6 out]
        n120 = call "ZK注射泵操作.vi"("是否启用通讯通知"=TRUE, "注射泵操作"=质控注射泵操作."关闭三通阀", "Slave ID"=w204) -> ("error out"=w207:errorcluster)  [unwired: 8 in]
      }
      event "注射泵注入": Value Change {
        n121 = event-data() -> ()  [unwired: 1 in, 6 out]
        n122 = Multiply(x=sgl 2.0, y="注射泵注入量") -> (x*y=w209:sgl)
        n123 = call "ZK注射泵操作.vi"("是否启用通讯通知"=FALSE, "注射泵操作"=质控注射泵操作."关闭三通阀", "Slave ID"=w210) -> ("error out"=w211:errorcluster)  [unwired: 8 in]
        n124 = call "ZK注射泵操作.vi"("是否启用通讯通知"=TRUE, "error in (no error)"=w211, "注射泵操作步"=w209, "注射泵操作"=质控注射泵操作."注射泵吸入", "Slave ID"=w210) -> ("error out"=w217:errorcluster)  [unwired: 6 in]
      }
      event "注射泵注出": Value Change {
        n125 = event-data() -> ()  [unwired: 1 in, 6 out]
        n126 = Multiply(x="注射泵注出量", y=sgl 2.0) -> (x*y=w219:sgl)
        n127 = call "ZK注射泵操作.vi"("是否启用通讯通知"=FALSE, "注射泵操作"=质控注射泵操作."打开三通阀", "Slave ID"=w221) -> ("error out"=w220:errorcluster)  [unwired: 8 in]
        n128 = call "ZK注射泵操作.vi"("是否启用通讯通知"=TRUE, "error in (no error)"=w220, "注射泵操作步"=w219, "注射泵操作"=质控注射泵操作."注射泵排出", "Slave ID"=w221) -> ("error out"=w227:errorcluster)  [unwired: 6 in]
      }
      event "注射泵暂停": Value Change {
        n129 = event-data() -> ()  [unwired: 1 in, 6 out]
        n130 = call "ZK注射泵操作.vi"("是否启用通讯通知"=TRUE, "注射泵操作"=质控注射泵操作."注射泵暂停", "Slave ID"=w228) -> ("error out"=w231:errorcluster)  [unwired: 8 in]
      }
      event "注射泵复位": Value Change {
        n131 = event-data() -> ()  [unwired: 1 in, 6 out]
        n132 = call "ZK注射泵操作.vi"("是否启用通讯通知"=TRUE, "注射泵操作"=质控注射泵操作."注射泵复位", "Slave ID"=w232) -> ("error out"=w235:errorcluster)  [unwired: 8 in]
      }
      event "三通阀1关闭": Value Change {
        w239 = u16 1 items=["打开三通阀", "关闭三通阀"] ("三通阀1操作")
        n133 = event-data() -> ()  [unwired: 1 in, 6 out]
        n134 = call "ZK三通阀1操作.vi"("是否启用通讯通知"=TRUE, "三通阀1操作"=w239, "Slave ID"=w236) -> ("error out"=w238:errorcluster)  [unwired: 8 in]
      }
      event "三通阀1打开": Value Change {
        w243 = u16 0 items=["打开三通阀", "关闭三通阀"] ("三通阀1操作")
        n135 = event-data() -> ()  [unwired: 1 in, 6 out]
        n136 = call "ZK三通阀1操作.vi"("是否启用通讯通知"=TRUE, "三通阀1操作"=w243, "Slave ID"=w240) -> ("error out"=w242:errorcluster)  [unwired: 8 in]
      }
      event "三通阀2打开": Value Change {
        w247 = u16 0 items=["打开三通阀", "关闭三通阀"] ("三通阀2操作")
        n137 = event-data() -> ()  [unwired: 1 in, 6 out]
        n138 = call "ZK三通阀2操作.vi"("是否启用通讯通知"=TRUE, "三通阀2操作"=w247, "Slave ID"=w244) -> ("error out"=w246:errorcluster)  [unwired: 8 in]
      }
      event "三通阀2关闭": Value Change {
        w251 = u16 1 items=["打开三通阀", "关闭三通阀"] ("三通阀2操作")
        n139 = event-data() -> ()  [unwired: 1 in, 6 out]
        n140 = call "ZK三通阀2操作.vi"("是否启用通讯通知"=TRUE, "三通阀2操作"=w251, "Slave ID"=w248) -> ("error out"=w250:errorcluster)  [unwired: 8 in]
      }
      event "蠕动泵1反转": Value Change {
        w254 = T11 3 items=["蠕动泵正转"=2, "蠕动泵反转"=3, "蠕动泵停止"=4] ("蠕动泵1操作")
        n141 = event-data() -> ()  [unwired: 1 in, 6 out]
        n142 = call "ZK蠕动泵1操作.vi"("是否启用通讯通知"=TRUE, "蠕动泵1操作"=w254, "Slave ID"=w252) -> ("error out"=w255:errorcluster)  [unwired: 8 in]
      }
      event "蠕动泵1正转": Value Change {
        w258 = T11 2 items=["蠕动泵正转"=2, "蠕动泵反转"=3, "蠕动泵停止"=4] ("蠕动泵1操作")
        n143 = event-data() -> ()  [unwired: 1 in, 6 out]
        n144 = call "ZK蠕动泵1操作.vi"("是否启用通讯通知"=TRUE, "蠕动泵1操作"=w258, "Slave ID"=w256) -> ("error out"=w259:errorcluster)  [unwired: 8 in]
      }
      event "蠕动泵1停止": Value Change {
        w262 = T11 4 items=["蠕动泵正转"=2, "蠕动泵反转"=3, "蠕动泵停止"=4] ("蠕动泵1操作")
        n145 = event-data() -> ()  [unwired: 1 in, 6 out]
        n146 = call "ZK蠕动泵1操作.vi"("是否启用通讯通知"=TRUE, "蠕动泵1操作"=w262, "Slave ID"=w260) -> ("error out"=w263:errorcluster)  [unwired: 8 in]
      }
      event "蠕动泵2反转": Value Change {
        w266 = T11 3 items=["蠕动泵正转"=2, "蠕动泵反转"=3, "蠕动泵停止"=4] ("蠕动泵2操作")
        n147 = event-data() -> ()  [unwired: 1 in, 6 out]
        n148 = call "ZK蠕动泵2操作.vi"("是否启用通讯通知"=TRUE, "蠕动泵2操作"=w266, "Slave ID"=w264) -> ("error out"=w267:errorcluster)  [unwired: 8 in]
      }
      event "蠕动泵2正转": Value Change {
        w270 = T11 2 items=["蠕动泵正转"=2, "蠕动泵反转"=3, "蠕动泵停止"=4] ("蠕动泵2操作")
        n149 = event-data() -> ()  [unwired: 1 in, 6 out]
        n150 = call "ZK蠕动泵2操作.vi"("是否启用通讯通知"=TRUE, "蠕动泵2操作"=w270, "Slave ID"=w268) -> ("error out"=w271:errorcluster)  [unwired: 8 in]
      }
      event "蠕动泵2停止": Value Change {
        w274 = T11 4 items=["蠕动泵正转"=2, "蠕动泵反转"=3, "蠕动泵停止"=4] ("蠕动泵2操作")
        n151 = event-data() -> ()  [unwired: 1 in, 6 out]
        n152 = call "ZK蠕动泵2操作.vi"("是否启用通讯通知"=TRUE, "蠕动泵2操作"=w274, "Slave ID"=w272) -> ("error out"=w275:errorcluster)  [unwired: 8 in]
      }
      event "组合操作进水样": Value Change {
        n153 = event-data() -> ()  [unwired: 1 in, 6 out]
        n154 = call "ZK组合命令区.vi"("是否启用通讯通知"=TRUE, "组合命令区"=质控组合命令区."进水样", "Slave ID"=w276) -> ("error out"=w279:errorcluster)  [unwired: 8 in]
      }
      event "组合操作排废液": Value Change {
        n155 = event-data() -> ()  [unwired: 1 in, 6 out]
        n156 = call "ZK组合命令区.vi"("是否启用通讯通知"=TRUE, "组合命令区"=质控组合命令区."排废液", "Slave ID"=w280) -> ("error out"=w283:errorcluster)  [unwired: 8 in]
      }
      event "组合操作进空气": Value Change {
        n157 = event-data() -> ()  [unwired: 1 in, 6 out]
        n158 = call "ZK组合命令区.vi"("是否启用通讯通知"=TRUE, "组合命令区"=质控组合命令区."进空气（搅拌）", "Slave ID"=w284) -> ("error out"=w287:errorcluster)  [unwired: 8 in]
      }
      event "组合操作定量": Value Change {
        n159 = event-data() -> ()  [unwired: 1 in, 6 out]
        n160 = call "ZK组合命令区.vi"("是否启用通讯通知"=TRUE, "组合命令区"=质控组合命令区."定量（反转定量）", "Slave ID"=w288) -> ("error out"=w291:errorcluster)  [unwired: 8 in]
      }
      event "组合操作加标": Value Change {
        n161 = event-data() -> ()  [unwired: 1 in, 6 out]
        n162 = call "ZK组合命令区.vi"("是否启用通讯通知"=TRUE, "加标体积"="加标体积输入", "组合命令区"=质控组合命令区."加标", "Slave ID"=w293) -> ("error out"=w296:errorcluster)  [unwired: 7 in]
      }
      event "组合操作停止": Value Change {
        n163 = event-data() -> ()  [unwired: 1 in, 6 out]
        n164 = call "ZK组合命令区.vi"("是否启用通讯通知"=TRUE, "组合命令区"=质控组合命令区."停止", "Slave ID"=w297) -> ("error out"=w300:errorcluster)  [unwired: 8 in]
      }
      event "启动进样流程": Value Change {
        n165 = event-data() -> ()  [unwired: 1 in, 6 out]
        n166 = call "ZK流程控制.vi"("是否启用通讯通知"=TRUE, "流程控制"=质控流程控制."启动进样流程", "Slave ID"=w301) -> ("error out"=w304:errorcluster)  [unwired: 8 in]
      }
      event "启动加标流程": Value Change {
        n167 = event-data() -> ()  [unwired: 1 in, 6 out]
        n168 = call "ZK流程控制.vi"("是否启用通讯通知"=TRUE, "流程控制"=质控流程控制."启动加标流程", "Slave ID"=w305) -> ("error out"=w308:errorcluster)  [unwired: 8 in]
      }
      event "启动排液流程": Value Change {
        n169 = event-data() -> ()  [unwired: 1 in, 6 out]
        n170 = call "ZK流程控制.vi"("是否启用通讯通知"=TRUE, "流程控制"=质控流程控制."启动排液流程", "Slave ID"=w309) -> ("error out"=w312:errorcluster)  [unwired: 8 in]
      }
      event "停止所有流程": Value Change {
        n171 = event-data() -> ()  [unwired: 1 in, 6 out]
        n172 = call "ZK流程控制.vi"("是否启用通讯通知"=TRUE, "流程控制"=质控流程控制."停止流程", "Slave ID"=w313) -> ("error out"=w316:errorcluster)  [unwired: 8 in]
      }
    }
  }
  n173 = property on="Tab Control 3" class="TabCtl (严格)"("Visible"=w1) -> ("Visible"=w8:bool)  [unwired: 2 in, 2 out]
  n174 = Select(t=T4 {"Left"=744, "Top"=804} ("位置"), s=w8, f=T4 {"Left"=744, "Top"=432} ("位置")) -> (s? t:f=w10:T4)
  n175 = Select(t=T4 {"Left"=900, "Top"=880} ("位置"), s=w8, f=T4 {"Left"=900, "Top"=500} ("位置")) -> (s? t:f=w5:T4)
  n176 = property class="App"() -> ("Disp.WkSpace"=w6:T12)  [unwired: 2 in, 2 out]
  n177 = property on="关闭" class="Bool"("Position"=w10) -> ()  [unwired: 2 in, 2 out]
  n178 = control-ref of="本VI"() -> (w3:refnum<vi>)
  n179 = call "取中心点.vi"("前面板窗口:最小尺寸"=w5, "显示:主工作区"=w6) -> ("前面板窗口:窗口边界"=w4:T12)  [unwired: 9 in]
  n180 = property class="VI"(reference=w3, "Front Panel.PanelBounds"=w4) -> ()  [unwired: 1 in, 2 out]
